vi "Build_Class_Tree.vi"() -> (2 "Root IDs":string[](array[string]), 3 "Map":map{string, cluster{string, variant}}(c390))   [LabVIEW 2025]
uses:
  <vilib>/_script/All Supported PropertiesOrMethods TypeDefs/ASC_ArrayOfUniqueIDStringParentIDStringName.ctl
  <vilib>/_script/All Supported PropertiesOrMethods TypeDefs/ASC_UniqueIDStringParentIDStringName.ctl
panel:
  out "size(s)":i32
  in  "All Types[]":T1=[{"Unique ID string"="3", "Parent ID string"="", "Class Name (unlocalized)"="Generic", "Class Name (localized)"="Generic"}, {"Unique ID string"="1", "Parent ID string"="", "Class Name (unlocalized)"="Application", "Class Name (localized)"="Application"}, {"Unique ID string"="2", "Parent ID string"="", "Class Name (unlocalized)"="VI", "Class Name (localized)"="VI"}, {"Unique ID string"="73", "Parent ID string"="", "Class Name (unlocalized)"="Project", "Class Name (localized)"="Project"}, {"Unique ID string"="74", "Parent ID string"="", "Class Name (unlocalized)"="ProjectItem", "Class Name (localized)"="ProjectItem"}, {"Unique ID string"="101", "Parent ID string"="2", "Class Name (unlocalized)"="PolymorphicVI", "Class Name (localized)"="PolymorphicVI"}, {"Unique ID string"="79", "Parent ID string"="2", "Class Name (unlocalized)"="FacadeVI", "Class Name (localized)"="FacadeVI"}, {"Unique ID string"="80", "Parent ID string"="74", "Class Name (unlocalized)"="Library", "Class Name (localized)"="Library"}, {"Unique ID string"="81", "Parent ID string"="", "Class Name (unlocalized)"="Variable", "Class Name (localized)"="Variable"}, {"Unique ID string"="82", "Parent ID string"="", "Class Name (unlocalized)"="TagSet", "Class Name (localized)"="TagSet"}, {"Unique ID string"="87", "Parent ID string"="2", "Class Name (unlocalized)"="MethodVI", "Class Name (localized)"="MethodVI"}, {"Unique ID string"="103", "Parent ID string"="80", "Class Name (unlocalized)"="XInterfaceLibrary", "Class Name (localized)"="XInterfaceLibrary"}, {"Unique ID string"="88", "Parent ID string"="103", "Class Name (unlocalized)"="XControlLibrary", "Class Name (localized)"="XControlLibrary"}, {"Unique ID string"="91", "Parent ID string"="", "Class Name (unlocalized)"="LVTarget", "Class Name (localized)"="LVTarget"}, {"Unique ID string"="93", "Parent ID string"="", "Class Name (unlocalized)"="Provider", "Class Name (localized)"="Provider"}, {"Unique ID string"="94", "Parent ID string"="", "Class Name (unlocalized)"="CopyOperation", "Class Name (localized)"="CopyOperation"}, {"Unique ID string"="95", "Parent ID string"="74", "Class Name (unlocalized)"="TargetItem", "Class Name (localized)"="TargetItem"}, {"Unique ID string"="96", "Parent ID string"="", "Class Name (unlocalized)"="ProjectItemType", "Class Name (localized)"="ProjectItemType"}, {"Unique ID string"="97", "Parent ID string"="", "Class Name (unlocalized)"="CopyItem", "Class Name (localized)"="CopyItem"}, {"Unique ID string"="98", "Parent ID string"="", "Class Name (unlocalized)"="CopyConflict", "Class Name (localized)"="CopyConflict"}, {"Unique ID string"="99", "Parent ID string"="", "Class Name (unlocalized)"="CopyExpert", "Class Name (localized)"="CopyExpert"}, {"Unique ID string"="123", "Parent ID string"="", "Class Name (unlocalized)"="Scene", "Class Name (localized)"="Scene"}, {"Unique ID string"="111", "Parent ID string"="123", "Class Name (unlocalized)"="SceneTexture", "Class Name (localized)"="SceneTexture"}, {"Unique ID string"="104", "Parent ID string"="123", "Class Name (unlocalized)"="SceneNode", "Class Name (localized)"="SceneNode"}, {"Unique ID string"="106", "Parent ID string"="104", "Class Name (unlocalized)"="SceneLight", "Class Name (localized)"="SceneLight"}, {"Unique ID string"="128", "Parent ID string"="123", "Class Name (unlocalized)"="SceneDrawable", "Class Name (localized)"="SceneDrawable"}, {"Unique ID string"="112", "Parent ID string"="128", "Class Name (unlocalized)"="SceneGeometry", "Class Name (localized)"="SceneGeometry"}, {"Unique ID string"="118", "Parent ID string"="112", "Class Name (unlocalized)"="SceneMesh", "Class Name (localized)"="SceneMesh"}, {"Unique ID string"="116", "Parent ID string"="112", "Class Name (unlocalized)"="SceneHeightField", "Class Name (localized)"="SceneHeightField"}, {"Unique ID string"="115", "Parent ID string"="112", "Class Name (unlocalized)"="SceneCylinder", "Class Name (localized)"="SceneCylinder"}, {"Unique ID string"="117", "Parent ID string"="112", "Class Name (unlocalized)"="SceneSphere", "Class Name (localized)"="SceneSphere"}, {"Unique ID string"="114", "Parent ID string"="112", "Class Name (unlocalized)"="SceneCone", "Class Name (localized)"="SceneCone"}, {"Unique ID string"="113", "Parent ID string"="112", "Class Name (unlocalized)"="SceneBox", "Class Name (localized)"="SceneBox"}, {"Unique ID string"="105", "Parent ID string"="104", "Class Name (unlocalized)"="SceneObject", "Class Name (localized)"="SceneObject"}, {"Unique ID string"="110", "Parent ID string"="104", "Class Name (unlocalized)"="SceneClipPlane", "Class Name (localized)"="SceneClipPlane"}, {"Unique ID string"="84", "Parent ID string"="123", "Class Name (unlocalized)"="SceneWindow", "Class Name (localized)"="SceneWindow"}, {"Unique ID string"="120", "Parent ID string"="74", "Class Name (unlocalized)"="PropertyFolder", "Class Name (localized)"="PropertyFolder"}, {"Unique ID string"="119", "Parent ID string"="120", "Class Name (unlocalized)"="XPropertyFolder", "Class Name (localized)"="XPropertyFolder"}, {"Unique ID string"="125", "Parent ID string"="74", "Class Name (unlocalized)"="LibraryData", "Class Name (localized)"="LibraryData"}, {"Unique ID string"="129", "Parent ID string"="128", "Class Name (unlocalized)"="SceneText", "Class Name (localized)"="SceneText"}, {"Unique ID string"="62", "Parent ID string"="2", "Class Name (unlocalized)"="SubsystemVI", "Class Name (localized)"="SubsystemVI"}, {"Unique ID string"="133", "Parent ID string"="", "Class Name (unlocalized)"="ProjectFilesViewItem", "Class Name (localized)"="ProjectFilesViewItem"}, {"Unique ID string"="134", "Parent ID string"="74", "Class Name (unlocalized)"="LVClassPropDefFolder", "Class Name (localized)"="LVClassPropDefFolder"}, {"Unique ID string"="36", "Parent ID string"="3", "Class Name (unlocalized)"="GObject", "Class Name (localized)"="GObject"}, {"Unique ID string"="37", "Parent ID string"="3", "Class Name (unlocalized)"="Plot", "Class Name (localized)"="Plot"}, {"Unique ID string"="38", "Parent ID string"="3", "Class Name (unlocalized)"="Cursor", "Class Name (localized)"="Cursor"}, {"Unique ID string"="4", "Parent ID string"="36", "Class Name (unlocalized)"="Decoration", "Class Name (localized)"="Decoration"}, {"Unique ID string"="5", "Parent ID string"="4", "Class Name (unlocalized)"="Text", "Class Name (localized)"="Text"}, {"Unique ID string"="39", "Parent ID string"="5", "Class Name (unlocalized)"="NumericText", "Class Name (localized)"="NumericText"}, {"Unique ID string"="40", "Parent ID string"="36", "Class Name (unlocalized)"="Scale", "Class Name (localized)"="Scale"}, {"Unique ID string"="41", "Parent ID string"="40", "Class Name (unlocalized)"="ColorScale", "Class Name (localized)"="ColorScale"}, {"Unique ID string"="42", "Parent ID string"="40", "Class Name (unlocalized)"="GraphScale", "Class Name (localized)"="GraphScale"}, {"Unique ID string"="43", "Parent ID string"="40", "Class Name (unlocalized)"="ColorGraphScale", "Class Name (localized)"="ColorGraphScale"}, {"Unique ID string"="6", "Parent ID string"="36", "Class Name (unlocalized)"="Control", "Class Name (localized)"="Control"}, {"Unique ID string"="7", "Parent ID string"="6", "Class Name (unlocalized)"="ColorBox", "Class Name (localized)"="ColorBox"}, {"Unique ID string"="8", "Parent ID string"="6", "Class Name (unlocalized)"="Boolean", "Class Name (localized)"="Boolean"}, {"Unique ID string"="9", "Parent ID string"="6", "Class Name (unlocalized)"="RefNum", "Class Name (localized)"="RefNum"}, {"Unique ID string"="44", "Parent ID string"="9", "Class Name (unlocalized)"="TypedRefNum", "Class Name (localized)"="TypedRefNum"}, {"Unique ID string"="10", "Parent ID string"="6", "Class Name (unlocalized)"="LVVariant", "Class Name (localized)"="LVVariant"}, {"Unique ID string"="11", "Parent ID string"="6", "Class Name (unlocalized)"="Path", "Class Name (localized)"="Path"}, {"Unique ID string"="12", "Parent ID string"="6", "Class Name (unlocalized)"="ListBox", "Class Name (localized)"="ListBox"}, {"Unique ID string"="13", "Parent ID string"="6", "Class Name (unlocalized)"="Table", "Class Name (localized)"="Table"}, {"Unique ID string"="14", "Parent ID string"="6", "Class Name (unlocalized)"="Array", "Class Name (localized)"="Array"}, {"Unique ID string"="15", "Parent ID string"="6", "Class Name (unlocalized)"="Picture", "Class Name (localized)"="Picture"}, {"Unique ID string"="16", "Parent ID string"="6", "Class Name (unlocalized)"="ActiveXContainer", "Class Name (localized)"="ActiveXContainer"}, {"Unique ID string"="17", "Parent ID string"="6", "Class Name (unlocalized)"="Numeric", "Class Name (localized)"="Numeric"}, {"Unique ID string"="18", "Parent ID string"="17", "Class Name (unlocalized)"="Digital", "Class Name (localized)"="Digital"}, {"Unique ID string"="19", "Parent ID string"="17", "Class Name (unlocalized)"="NamedNumeric", "Class Name (localized)"="NamedNumeric"}, {"Unique ID string"="35", "Parent ID string"="19", "Class Name (unlocalized)"="Enum", "Class Name (localized)"="Enum"}, {"Unique ID string"="34", "Parent ID string"="19", "Class Name (unlocalized)"="Ring", "Class Name (localized)"="Ring"}, {"Unique ID string"="20", "Parent ID string"="17", "Class Name (unlocalized)"="ColorRamp", "Class Name (localized)"="ColorRamp"}, {"Unique ID string"="33", "Parent ID string"="17", "Class Name (unlocalized)"="NumericWithScale", "Class Name (localized)"="NumericWithScale"}, {"Unique ID string"="21", "Parent ID string"="33", "Class Name (unlocalized)"="Slide", "Class Name (localized)"="Slide"}, {"Unique ID string"="32", "Parent ID string"="33", "Class Name (unlocalized)"="Knob", "Class Name (localized)"="Knob"}, {"Unique ID string"="22", "Parent ID string"="6", "Class Name (unlocalized)"="GraphChart", "Class Name (localized)"="GraphChart"}, {"Unique ID string"="23", "Parent ID string"="22", "Class Name (unlocalized)"="WaveformChart", "Class Name (localized)"="WaveformChart"}, {"Unique ID string"="24", "Parent ID string"="22", "Class Name (unlocalized)"="WaveformGraph", "Class Name (localized)"="WaveformGraph"}, {"Unique ID string"="25", "Parent ID string"="22", "Class Name (unlocalized)"="IntensityChart", "Class Name (localized)"="IntensityChart"}, {"Unique ID string"="26", "Parent ID string"="22", "Class Name (unlocalized)"="IntensityGraph", "Class Name (localized)"="IntensityGraph"}, {"Unique ID string"="27", "Parent ID string"="6", "Class Name (unlocalized)"="String", "Class Name (localized)"="String"}, {"Unique ID string"="28", "Parent ID string"="6", "Class Name (unlocalized)"="IOName", "Class Name (localized)"="IOName"}, {"Unique ID string"="29", "Parent ID string"="27", "Class Name (unlocalized)"="ComboBox", "Class Name (localized)"="ComboBox"}, {"Unique ID string"="30", "Parent ID string"="6", "Class Name (unlocalized)"="Cluster", "Class Name (localized)"="Cluster"}, {"Unique ID string"="31", "Parent ID string"="36", "Class Name (unlocalized)"="Panel", "Class Name (localized)"="Panel"}, {"Unique ID string"="46", "Parent ID string"="6", "Class Name (unlocalized)"="MulticolumnListbox", "Class Name (localized)"="MulticolumnListbox"}, {"Unique ID string"="47", "Parent ID string"="6", "Class Name (unlocalized)"="WaveformData", "Class Name (localized)"="WaveformData"}, {"Unique ID string"="48", "Parent ID string"="28", "Class Name (unlocalized)"="DSCTag", "Class Name (localized)"="DSCTag"}, {"Unique ID string"="49", "Parent ID string"="28", "Class Name (unlocalized)"="DAQChannelName", "Class Name (localized)"="DAQChannelName"}, {"Unique ID string"="50", "Parent ID string"="28", "Class Name (unlocalized)"="VISAResourceName", "Class Name (localized)"="VISAResourceName"}, {"Unique ID string"="51", "Parent ID string"="28", "Class Name (unlocalized)"="IVILogicalName", "Class Name (localized)"="IVILogicalName"}, {"Unique ID string"="52", "Parent ID string"="40", "Class Name (unlocalized)"="SlideScale", "Class Name (localized)"="SlideScale"}, {"Unique ID string"="53", "Parent ID string"="6", "Class Name (unlocalized)"="PageSelector", "Class Name (localized)"="PageSelector"}, {"Unique ID string"="54", "Parent ID string"="3", "Class Name (unlocalized)"="Page", "Class Name (localized)"="Page"}, {"Unique ID string"="55", "Parent ID string"="53", "Class Name (unlocalized)"="TabControl", "Class Name (localized)"="TabControl"}, {"Unique ID string"="56", "Parent ID string"="3", "Class Name (unlocalized)"="ConnectorPane", "Class Name (localized)"="ConnectorPane"}, {"Unique ID string"="57", "Parent ID string"="28", "Class Name (unlocalized)"="DAQmxName", "Class Name (localized)"="DAQmxName"}, {"Unique ID string"="59", "Parent ID string"="9", "Class Name (unlocalized)"="LVObjectRefNum", "Class Name (localized)"="LVObjectRefNum"}, {"Unique ID string"="58", "Parent ID string"="59", "Class Name (unlocalized)"="VIRefNum", "Class Name (localized)"="VIRefNum"}, {"Unique ID string"="60", "Parent ID string"="6", "Class Name (unlocalized)"="AbsTime", "Class Name (localized)"="AbsTime"}, {"Unique ID string"="61", "Parent ID string"="6", "Class Name (unlocalized)"="DigitalTable", "Class Name (localized)"="DigitalTable"}, {"Unique ID string"="66", "Parent ID string"="6", "Class Name (unlocalized)"="TreeControl", "Class Name (localized)"="TreeControl"}, {"Unique ID string"="67", "Parent ID string"="28", "Class Name (unlocalized)"="GenClassTagRef", "Class Name (localized)"="GenClassTagRef"}, {"Unique ID string"="68", "Parent ID string"="9", "Class Name (unlocalized)"="GenClassRef", "Class Name (localized)"="GenClassRef"}, {"Unique ID string"="65", "Parent ID string"="6", "Class Name (unlocalized)"="SubPanel", "Class Name (localized)"="SubPanel"}, {"Unique ID string"="69", "Parent ID string"="41", "Class Name (unlocalized)"="RotaryColorScale", "Class Name (localized)"="RotaryColorScale"}, {"Unique ID string"="70", "Parent ID string"="6", "Class Name (unlocalized)"="PlugInControl", "Class Name (localized)"="PlugInControl"}, {"Unique ID string"="71", "Parent ID string"="6", "Class Name (unlocalized)"="PlugInDDODummyContainer", "Class Name (localized)"="PlugInDDODummyContainer"}, {"Unique ID string"="122", "Parent ID string"="28", "Class Name (unlocalized)"="GenClassTagFlatRef", "Class Name (localized)"="GenClassTagFlatRef"}, {"Unique ID string"="72", "Parent ID string"="30", "Class Name (unlocalized)"="RadioButtonsControl", "Class Name (localized)"="RadioButtonsControl"}, {"Unique ID string"="75", "Parent ID string"="36", "Class Name (unlocalized)"="Pane", "Class Name (localized)"="Pane"}, {"Unique ID string"="77", "Parent ID string"="74", "Class Name (unlocalized)"="BuildSpecification", "Class Name (localized)"="BuildSpecification"}, {"Unique ID string"="78", "Parent ID string"="6", "Class Name (unlocalized)"="Pixmap", "Class Name (localized)"="Pixmap"}, {"Unique ID string"="83", "Parent ID string"="24", "Class Name (unlocalized)"="XYGraph", "Class Name (localized)"="XYGraph"}, {"Unique ID string"="76", "Parent ID string"="36", "Class Name (unlocalized)"="Splitter", "Class Name (localized)"="Splitter"}, {"Unique ID string"="85", "Parent ID string"="80", "Class Name (unlocalized)"="LVClassLibrary", "Class Name (localized)"="LVClassLibrary"}, {"Unique ID string"="89", "Parent ID string"="103", "Class Name (unlocalized)"="XNodeLibrary", "Class Name (localized)"="XNodeLibrary"}, {"Unique ID string"="90", "Parent ID string"="6", "Class Name (unlocalized)"="Scrollbar", "Class Name (localized)"="Scrollbar"}, {"Unique ID string"="92", "Parent ID string"="22", "Class Name (unlocalized)"="MixedSignalGraph", "Class Name (localized)"="MixedSignalGraph"}, {"Unique ID string"="100", "Parent ID string"="6", "Class Name (unlocalized)"="SceneGraphDisplay", "Class Name (localized)"="SceneGraphDisplay"}, {"Unique ID string"="102", "Parent ID string"="6", "Class Name (unlocalized)"="LabVIEWClassControl", "Class Name (localized)"="LabVIEWClassControl"}, {"Unique ID string"="121", "Parent ID string"="24", "Class Name (unlocalized)"="DigitalGraph", "Class Name (localized)"="DigitalGraph"}, {"Unique ID string"="126", "Parent ID string"="80", "Class Name (unlocalized)"="StatechartLibrary", "Class Name (localized)"="StatechartLibrary"}, {"Unique ID string"="127", "Parent ID string"="6", "Class Name (unlocalized)"="MixedCheckbox", "Class Name (localized)"="MixedCheckbox"}, {"Unique ID string"="130", "Parent ID string"="6", "Class Name (unlocalized)"="MultiSegmentPipe", "Class Name (localized)"="MultiSegmentPipe"}, {"Unique ID string"="131", "Parent ID string"="3", "Class Name (unlocalized)"="Bus", "Class Name (localized)"="Bus"}, {"Unique ID string"="132", "Parent ID string"="6", "Class Name (unlocalized)"="StubDDO", "Class Name (localized)"="StubDDO"}, {"Unique ID string"="135", "Parent ID string"="44", "Class Name (unlocalized)"="DataValRefNum", "Class Name (localized)"="DataValRefNum"}, {"Unique ID string"="136", "Parent ID string"="6", "Class Name (unlocalized)"="Set", "Class Name (localized)"="Set"}, {"Unique ID string"="137", "Parent ID string"="6", "Class Name (unlocalized)"="Map", "Class Name (localized)"="Map"}, {"Unique ID string"="16503", "Parent ID string"="36", "Class Name (unlocalized)"="AbstractDiagram", "Class Name (localized)"="AbstractDiagram"}, {"Unique ID string"="16384", "Parent ID string"="16503", "Class Name (unlocalized)"="Diagram", "Class Name (localized)"="Diagram"}, {"Unique ID string"="16423", "Parent ID string"="16384", "Class Name (unlocalized)"="TopLevelDiagram", "Class Name (localized)"="TopLevelDiagram"}, {"Unique ID string"="16385", "Parent ID string"="36", "Class Name (unlocalized)"="Terminal", "Class Name (localized)"="Terminal"}, {"Unique ID string"="16386", "Parent ID string"="36", "Class Name (unlocalized)"="Constant", "Class Name (localized)"="Constant"}, {"Unique ID string"="16387", "Parent ID string"="16386", "Class Name (unlocalized)"="PathConstant", "Class Name (localized)"="PathConstant"}, {"Unique ID string"="16388", "Parent ID string"="16386", "Class Name (unlocalized)"="ArrayConstant", "Class Name (localized)"="ArrayConstant"}, {"Unique ID string"="16389", "Parent ID string"="16386", "Class Name (unlocalized)"="NumericConstant", "Class Name (localized)"="NumericConstant"}, {"Unique ID string"="16390", "Parent ID string"="16389", "Class Name (unlocalized)"="DigitalNumericConstant", "Class Name (localized)"="DigitalNumericConstant"}, {"Unique ID string"="16391", "Parent ID string"="16389", "Class Name (unlocalized)"="NamedNumericConstant", "Class Name (localized)"="NamedNumericConstant"}, {"Unique ID string"="16424", "Parent ID string"="16391", "Class Name (unlocalized)"="RingConstant", "Class Name (localized)"="RingConstant"}, {"Unique ID string"="16425", "Parent ID string"="16391", "Class Name (unlocalized)"="EnumConstant", "Class Name (localized)"="EnumConstant"}, {"Unique ID string"="16392", "Parent ID string"="16386", "Class Name (unlocalized)"="StringConstant", "Class Name (localized)"="StringConstant"}, {"Unique ID string"="16393", "Parent ID string"="16386", "Class Name (unlocalized)"="ClusterConstant", "Class Name (localized)"="ClusterConstant"}, {"Unique ID string"="16394", "Parent ID string"="16386", "Class Name (unlocalized)"="FixedConstant", "Class Name (localized)"="FixedConstant"}, {"Unique ID string"="16422", "Parent ID string"="16386", "Class Name (unlocalized)"="BooleanConstant", "Class Name (localized)"="BooleanConstant"}, {"Unique ID string"="16395", "Parent ID string"="16385", "Class Name (unlocalized)"="ControlTerminal", "Class Name (localized)"="ControlTerminal"}, {"Unique ID string"="16396", "Parent ID string"="36", "Class Name (unlocalized)"="FormulaParameter", "Class Name (localized)"="FormulaParameter"}, {"Unique ID string"="16426", "Parent ID string"="36", "Class Name (unlocalized)"="Tunnel", "Class Name (localized)"="Tunnel"}, {"Unique ID string"="16427", "Parent ID string"="16426", "Class Name (unlocalized)"="LoopTunnel", "Class Name (localized)"="LoopTunnel"}, {"Unique ID string"="16399", "Parent ID string"="16426", "Class Name (unlocalized)"="RightShiftRegister", "Class Name (localized)"="RightShiftRegister"}, {"Unique ID string"="16428", "Parent ID string"="36", "Class Name (unlocalized)"="SequenceLocal", "Class Name (localized)"="SequenceLocal"}, {"Unique ID string"="16421", "Parent ID string"="36", "Class Name (unlocalized)"="Node", "Class Name (localized)"="Node"}, {"Unique ID string"="16397", "Parent ID string"="16421", "Class Name (unlocalized)"="Global", "Class Name (localized)"="Global"}, {"Unique ID string"="16398", "Parent ID string"="16421", "Class Name (unlocalized)"="Local", "Class Name (localized)"="Local"}, {"Unique ID string"="16400", "Parent ID string"="16421", "Class Name (unlocalized)"="Function", "Class Name (localized)"="Function"}, {"Unique ID string"="16429", "Parent ID string"="16400", "Class Name (unlocalized)"="Comparison", "Class Name (localized)"="Comparison"}, {"Unique ID string"="16430", "Parent ID string"="16400", "Class Name (unlocalized)"="ReadWriteFile", "Class Name (localized)"="ReadWriteFile"}, {"Unique ID string"="16431", "Parent ID string"="16400", "Class Name (unlocalized)"="TypeCast", "Class Name (localized)"="TypeCast"}, {"Unique ID string"="16432", "Parent ID string"="16400", "Class Name (unlocalized)"="FlattenUnflattenString", "Class Name (localized)"="FlattenUnflattenString"}, {"Unique ID string"="16433", "Parent ID string"="16400", "Class Name (unlocalized)"="GPIBReadWrite", "Class Name (localized)"="GPIBReadWrite"}, {"Unique ID string"="16401", "Parent ID string"="16421", "Class Name (unlocalized)"="SubVI", "Class Name (localized)"="SubVI"}, {"Unique ID string"="16402", "Parent ID string"="16421", "Class Name (unlocalized)"="CallByRef", "Class Name (localized)"="CallByRef"}, {"Unique ID string"="16403", "Parent ID string"="16421", "Class Name (unlocalized)"="UnitCast", "Class Name (localized)"="UnitCast"}, {"Unique ID string"="16404", "Parent ID string"="16421", "Class Name (unlocalized)"="Structure", "Class Name (localized)"="Structure"}, {"Unique ID string"="16405", "Parent ID string"="16404", "Class Name (unlocalized)"="Loop", "Class Name (localized)"="Loop"}, {"Unique ID string"="16434", "Parent ID string"="16405", "Class Name (unlocalized)"="ForLoop", "Class Name (localized)"="ForLoop"}, {"Unique ID string"="16435", "Parent ID string"="16405", "Class Name (unlocalized)"="WhileLoop", "Class Name (localized)"="WhileLoop"}, {"Unique ID string"="16406", "Parent ID string"="16404", "Class Name (unlocalized)"="MultiFrameStructure", "Class Name (localized)"="MultiFrameStructure"}, {"Unique ID string"="16407", "Parent ID string"="16406", "Class Name (unlocalized)"="Sequence", "Class Name (localized)"="Sequence"}, {"Unique ID string"="16408", "Parent ID string"="16406", "Class Name (unlocalized)"="CaseStructure", "Class Name (localized)"="CaseStructure"}, {"Unique ID string"="16409", "Parent ID string"="16421", "Class Name (unlocalized)"="Formula", "Class Name (localized)"="Formula"}, {"Unique ID string"="16436", "Parent ID string"="16409", "Class Name (unlocalized)"="ScriptNode", "Class Name (localized)"="ScriptNode"}, {"Unique ID string"="16437", "Parent ID string"="16400", "Class Name (unlocalized)"="ArrayToCluster", "Class Name (localized)"="ArrayToCluster"}, {"Unique ID string"="16410", "Parent ID string"="16421", "Class Name (unlocalized)"="GrowableFunction", "Class Name (localized)"="GrowableFunction"}, {"Unique ID string"="16411", "Parent ID string"="16410", "Class Name (unlocalized)"="BuildClusterArray", "Class Name (localized)"="BuildClusterArray"}, {"Unique ID string"="16412", "Parent ID string"="16410", "Class Name (unlocalized)"="CompoundArithmetic", "Class Name (localized)"="CompoundArithmetic"}, {"Unique ID string"="16413", "Parent ID string"="16410", "Class Name (unlocalized)"="IndexArray", "Class Name (localized)"="IndexArray"}, {"Unique ID string"="16416", "Parent ID string"="16410", "Class Name (unlocalized)"="CIN", "Class Name (localized)"="CIN"}, {"Unique ID string"="16417", "Parent ID string"="16410", "Class Name (unlocalized)"="CallLibrary", "Class Name (localized)"="CallLibrary"}, {"Unique ID string"="16438", "Parent ID string"="16410", "Class Name (unlocalized)"="FormatScanString", "Class Name (localized)"="FormatScanString"}, {"Unique ID string"="16418", "Parent ID string"="16410", "Class Name (unlocalized)"="ObjectFunction", "Class Name (localized)"="ObjectFunction"}, {"Unique ID string"="16419", "Parent ID string"="16418", "Class Name (unlocalized)"="Property", "Class Name (localized)"="Property"}, {"Unique ID string"="16420", "Parent ID string"="16418", "Class Name (unlocalized)"="Invoke", "Class Name (localized)"="Invoke"}, {"Unique ID string"="16439", "Parent ID string"="36", "Class Name (unlocalized)"="Wire", "Class Name (localized)"="Wire"}, {"Unique ID string"="16440", "Parent ID string"="3", "Class Name (unlocalized)"="Probe", "Class Name (localized)"="Probe"}, {"Unique ID string"="16441", "Parent ID string"="16385", "Class Name (unlocalized)"="InnerTerminal", "Class Name (localized)"="InnerTerminal"}, {"Unique ID string"="16442", "Parent ID string"="16426", "Class Name (unlocalized)"="LeftShiftRegister", "Class Name (localized)"="LeftShiftRegister"}, {"Unique ID string"="16443", "Parent ID string"="16401", "Class Name (unlocalized)"="PolymorphicSubVI", "Class Name (localized)"="PolymorphicSubVI"}, {"Unique ID string"="16444", "Parent ID string"="36", "Class Name (unlocalized)"="PropertyItem", "Class Name (localized)"="PropertyItem"}, {"Unique ID string"="16445", "Parent ID string"="16386", "Class Name (unlocalized)"="IONameConstant", "Class Name (localized)"="IONameConstant"}, {"Unique ID string"="16446", "Parent ID string"="16445", "Class Name (unlocalized)"="DSCTagConstant", "Class Name (localized)"="DSCTagConstant"}, {"Unique ID string"="16447", "Parent ID string"="16445", "Class Name (unlocalized)"="DAQChannelNameConstant", "Class Name (localized)"="DAQChannelNameConstant"}, {"Unique ID string"="16448", "Parent ID string"="16445", "Class Name (unlocalized)"="VISAResourceNameConstant", "Class Name (localized)"="VISAResourceNameConstant"}, {"Unique ID string"="16449", "Parent ID string"="16445", "Class Name (unlocalized)"="IVILogicalNameConstant", "Class Name (localized)"="IVILogicalNameConstant"}, {"Unique ID string"="16450", "Parent ID string"="16386", "Class Name (unlocalized)"="ColorBoxConstant", "Class Name (localized)"="ColorBoxConstant"}, {"Unique ID string"="16451", "Parent ID string"="16421", "Class Name (unlocalized)"="ControlReferenceConstant", "Class Name (localized)"="ControlReferenceConstant"}, {"Unique ID string"="16453", "Parent ID string"="16401", "Class Name (unlocalized)"="ConfNode", "Class Name (localized)"="ConfNode"}, {"Unique ID string"="16456", "Parent ID string"="16385", "Class Name (unlocalized)"="OuterTerminal", "Class Name (localized)"="OuterTerminal"}, {"Unique ID string"="16457", "Parent ID string"="16445", "Class Name (unlocalized)"="DAQmxNameConstant", "Class Name (localized)"="DAQmxNameConstant"}, {"Unique ID string"="16458", "Parent ID string"="16406", "Class Name (unlocalized)"="EventStructure", "Class Name (localized)"="EventStructure"}, {"Unique ID string"="16459", "Parent ID string"="36", "Class Name (unlocalized)"="FlatSequence", "Class Name (localized)"="FlatSequence"}, {"Unique ID string"="16460", "Parent ID string"="16445", "Class Name (unlocalized)"="GenClassTagRefConstant", "Class Name (localized)"="GenClassTagRefConstant"}, {"Unique ID string"="16461", "Parent ID string"="16386", "Class Name (unlocalized)"="AbsTimeConstant", "Class Name (localized)"="AbsTimeConstant"}, {"Unique ID string"="16462", "Parent ID string"="16407", "Class Name (unlocalized)"="ExternalNode", "Class Name (localized)"="ExternalNode"}, {"Unique ID string"="16466", "Parent ID string"="16392", "Class Name (unlocalized)"="ComboBoxConstant", "Class Name (localized)"="ComboBoxConstant"}, {"Unique ID string"="16463", "Parent ID string"="3", "Class Name (unlocalized)"="SubWizard", "Class Name (localized)"="SubWizard"}, {"Unique ID string"="16455", "Parent ID string"="16463", "Class Name (unlocalized)"="StateDiagramWizard", "Class Name (localized)"="StateDiagramWizard"}, {"Unique ID string"="16464", "Parent ID string"="16396", "Class Name (unlocalized)"="ScriptNodeParameter", "Class Name (localized)"="ScriptNodeParameter"}, {"Unique ID string"="16465", "Parent ID string"="16421", "Class Name (unlocalized)"="StaticVIReference", "Class Name (localized)"="StaticVIReference"}, {"Unique ID string"="16467", "Parent ID string"="16435", "Class Name (unlocalized)"="TimedLoop", "Class Name (localized)"="TimedLoop"}, {"Unique ID string"="16470", "Parent ID string"="16445", "Class Name (unlocalized)"="GenClassTagFlatRefConstant", "Class Name (localized)"="GenClassTagFlatRefConstant"}, {"Unique ID string"="16472", "Parent ID string"="16384", "Class Name (unlocalized)"="SimDiagram", "Class Name (localized)"="SimDiagram"}, {"Unique ID string"="16473", "Parent ID string"="16384", "Class Name (unlocalized)"="CompanionDiagram", "Class Name (localized)"="CompanionDiagram"}, {"Unique ID string"="16474", "Parent ID string"="16404", "Class Name (unlocalized)"="SimulationNode", "Class Name (localized)"="SimulationNode"}, {"Unique ID string"="16476", "Parent ID string"="16410", "Class Name (unlocalized)"="Bundler", "Class Name (localized)"="Bundler"}, {"Unique ID string"="16477", "Parent ID string"="16410", "Class Name (unlocalized)"="Unbundler", "Class Name (localized)"="Unbundler"}, {"Unique ID string"="16414", "Parent ID string"="16476", "Class Name (unlocalized)"="BuildArray", "Class Name (localized)"="BuildArray"}, {"Unique ID string"="16415", "Parent ID string"="16476", "Class Name (unlocalized)"="NamedBundler", "Class Name (localized)"="NamedBundler"}, {"Unique ID string"="16475", "Parent ID string"="36", "Class Name (unlocalized)"="SimulationDCO", "Class Name (localized)"="SimulationDCO"}, {"Unique ID string"="16478", "Parent ID string"="16477", "Class Name (unlocalized)"="NamedUnbundler", "Class Name (localized)"="NamedUnbundler"}, {"Unique ID string"="16479", "Parent ID string"="3", "Class Name (unlocalized)"="FlatSequenceFrame", "Class Name (localized)"="FlatSequenceFrame"}, {"Unique ID string"="16480", "Parent ID string"="36", "Class Name (unlocalized)"="FlatSequenceInnerTunnel", "Class Name (localized)"="FlatSequenceInnerTunnel"}, {"Unique ID string"="16481", "Parent ID string"="36", "Class Name (unlocalized)"="FlatSequenceOuterTunnel", "Class Name (localized)"="FlatSequenceOuterTunnel"}, {"Unique ID string"="16482", "Parent ID string"="16386", "Class Name (unlocalized)"="RefNumConstant", "Class Name (localized)"="RefNumConstant"}, {"Unique ID string"="16452", "Parent ID string"="16482", "Class Name (unlocalized)"="ClassSpecifierConstant", "Class Name (localized)"="ClassSpecifierConstant"}, {"Unique ID string"="16483", "Parent ID string"="16432", "Class Name (unlocalized)"="FlattenString", "Class Name (localized)"="FlattenString"}, {"Unique ID string"="16484", "Parent ID string"="36", "Class Name (unlocalized)"="PolymorphicVISelector", "Class Name (localized)"="PolymorphicVISelector"}, {"Unique ID string"="16485", "Parent ID string"="16421", "Class Name (unlocalized)"="XNode", "Class Name (localized)"="XNode"}, {"Unique ID string"="16486", "Parent ID string"="16525", "Class Name (unlocalized)"="SelectorTunnel", "Class Name (localized)"="SelectorTunnel"}, {"Unique ID string"="16487", "Parent ID string"="16406", "Class Name (unlocalized)"="DisableStructure", "Class Name (localized)"="DisableStructure"}, {"Unique ID string"="16491", "Parent ID string"="36", "Class Name (unlocalized)"="SynchronousDataFlowDCO", "Class Name (localized)"="SynchronousDataFlowDCO"}, {"Unique ID string"="16490", "Parent ID string"="16404", "Class Name (unlocalized)"="SynchronousDataFlowNode", "Class Name (localized)"="SynchronousDataFlowNode"}, {"Unique ID string"="16489", "Parent ID string"="16384", "Class Name (unlocalized)"="SDF Companion Diagram", "Class Name (localized)"="SDF Companion Diagram"}, {"Unique ID string"="16488", "Parent ID string"="16384", "Class Name (unlocalized)"="SDFDiagram", "Class Name (localized)"="SDFDiagram"}, {"Unique ID string"="16492", "Parent ID string"="16400", "Class Name (unlocalized)"="FileDialog", "Class Name (localized)"="FileDialog"}, {"Unique ID string"="16498", "Parent ID string"="16463", "Class Name (unlocalized)"="CodeWizard", "Class Name (localized)"="CodeWizard"}, {"Unique ID string"="16454", "Parent ID string"="3", "Class Name (unlocalized)"="MasterWizard", "Class Name (localized)"="MasterWizard"}, {"Unique ID string"="16494", "Parent ID string"="16479", "Class Name (unlocalized)"="TimeSequenceFrame", "Class Name (localized)"="TimeSequenceFrame"}, {"Unique ID string"="16495", "Parent ID string"="16459", "Class Name (unlocalized)"="TimeFlatSequence", "Class Name (localized)"="TimeFlatSequence"}, {"Unique ID string"="16496", "Parent ID string"="16404", "Class Name (unlocalized)"="TimedSequence", "Class Name (localized)"="TimedSequence"}, {"Unique ID string"="16493", "Parent ID string"="36", "Class Name (unlocalized)"="TimedStructDCO", "Class Name (localized)"="TimedStructDCO"}, {"Unique ID string"="16497", "Parent ID string"="16485", "Class Name (unlocalized)"="XDataNode", "Class Name (localized)"="XDataNode"}, {"Unique ID string"="16499", "Parent ID string"="16409", "Class Name (unlocalized)"="MathScriptNode", "Class Name (localized)"="MathScriptNode"}, {"Unique ID string"="16500", "Parent ID string"="16396", "Class Name (unlocalized)"="MathScriptNodeParameter", "Class Name (localized)"="MathScriptNodeParameter"}, {"Unique ID string"="16501", "Parent ID string"="16386", "Class Name (unlocalized)"="LabVIEWClassConstant", "Class Name (localized)"="LabVIEWClassConstant"}, {"Unique ID string"="16502", "Parent ID string"="16503", "Class Name (unlocalized)"="MathDiagram", "Class Name (localized)"="MathDiagram"}, {"Unique ID string"="16505", "Parent ID string"="16418", "Class Name (unlocalized)"="Constructor", "Class Name (localized)"="Constructor"}, {"Unique ID string"="16537", "Parent ID string"="16404", "Class Name (unlocalized)"="StatechartStructureNode", "Class Name (localized)"="StatechartStructureNode"}, {"Unique ID string"="16510", "Parent ID string"="16537", "Class Name (unlocalized)"="JoinNode", "Class Name (localized)"="JoinNode"}, {"Unique ID string"="16509", "Parent ID string"="16537", "Class Name (unlocalized)"="ForkNode", "Class Name (localized)"="ForkNode"}, {"Unique ID string"="16508", "Parent ID string"="16537", "Class Name (unlocalized)"="StateNode", "Class Name (localized)"="StateNode"}, {"Unique ID string"="16507", "Parent ID string"="16537", "Class Name (unlocalized)"="JunctionNode", "Class Name (localized)"="JunctionNode"}, {"Unique ID string"="16506", "Parent ID string"="16537", "Class Name (unlocalized)"="RegionNode", "Class Name (localized)"="RegionNode"}, {"Unique ID string"="16511", "Parent ID string"="16384", "Class Name (unlocalized)"="ScDiagram", "Class Name (localized)"="ScDiagram"}, {"Unique ID string"="16512", "Parent ID string"="16421", "Class Name (unlocalized)"="SharedVariableNode", "Class Name (localized)"="SharedVariableNode"}, {"Unique ID string"="16514", "Parent ID string"="16385", "Class Name (unlocalized)"="ParameterTerminal", "Class Name (localized)"="ParameterTerminal"}, {"Unique ID string"="16515", "Parent ID string"="16514", "Class Name (unlocalized)"="OverridableParameterTerminal", "Class Name (localized)"="OverridableParameterTerminal"}, {"Unique ID string"="16516", "Parent ID string"="16404", "Class Name (unlocalized)"="InPlaceElementStructure", "Class Name (localized)"="InPlaceElementStructure"}, {"Unique ID string"="16517", "Parent ID string"="16421", "Class Name (unlocalized)"="InPlaceBorderNode", "Class Name (localized)"="InPlaceBorderNode"}, {"Unique ID string"="16521", "Parent ID string"="16517", "Class Name (unlocalized)"="InPlaceElementNode", "Class Name (localized)"="InPlaceElementNode"}, {"Unique ID string"="16520", "Parent ID string"="16517", "Class Name (unlocalized)"="InPlaceVariantNode", "Class Name (localized)"="InPlaceVariantNode"}, {"Unique ID string"="16518", "Parent ID string"="16517", "Class Name (unlocalized)"="InPlaceArrayNode", "Class Name (localized)"="InPlaceArrayNode"}, {"Unique ID string"="16519", "Parent ID string"="16517", "Class Name (unlocalized)"="InPlaceClusterNode", "Class Name (localized)"="InPlaceClusterNode"}, {"Unique ID string"="16522", "Parent ID string"="16421", "Class Name (unlocalized)"="FeedbackNode", "Class Name (localized)"="FeedbackNode"}, {"Unique ID string"="16523", "Parent ID string"="16421", "Class Name (unlocalized)"="MathScriptCallByRef", "Class Name (localized)"="MathScriptCallByRef"}, {"Unique ID string"="16524", "Parent ID string"="16517", "Class Name (unlocalized)"="InPlaceDataValRefNode", "Class Name (localized)"="InPlaceDataValRefNode"}, {"Unique ID string"="16525", "Parent ID string"="16426", "Class Name (unlocalized)"="ConditionalTunnel", "Class Name (localized)"="ConditionalTunnel"}, {"Unique ID string"="16526", "Parent ID string"="16401", "Class Name (unlocalized)"="AbstractDynamicDispatch", "Class Name (localized)"="AbstractDynamicDispatch"}, {"Unique ID string"="16527", "Parent ID string"="16526", "Class Name (unlocalized)"="DynamicDispatchSubVI", "Class Name (localized)"="DynamicDispatchSubVI"}, {"Unique ID string"="16528", "Parent ID string"="16526", "Class Name (unlocalized)"="CallParentNode", "Class Name (localized)"="CallParentNode"}, {"Unique ID string"="16504", "Parent ID string"="16409", "Class Name (unlocalized)"="InlineCNode", "Class Name (localized)"="InlineCNode"}, {"Unique ID string"="16529", "Parent ID string"="16482", "Class Name (unlocalized)"="GenClassRefConst", "Class Name (localized)"="GenClassRefConst"}, {"Unique ID string"="16530", "Parent ID string"="16517", "Class Name (unlocalized)"="InPlaceArraySplitNode", "Class Name (localized)"="InPlaceArraySplitNode"}, {"Unique ID string"="16531", "Parent ID string"="16421", "Class Name (unlocalized)"="SharedVariableDynamicOpen", "Class Name (localized)"="SharedVariableDynamicOpen"}, {"Unique ID string"="16532", "Parent ID string"="16421", "Class Name (unlocalized)"="SharedVariableDynamicRead", "Class Name (localized)"="SharedVariableDynamicRead"}, {"Unique ID string"="16533", "Parent ID string"="16421", "Class Name (unlocalized)"="SharedVariableDynamicWrite", "Class Name (localized)"="SharedVariableDynamicWrite"}, {"Unique ID string"="16534", "Parent ID string"="16401", "Class Name (unlocalized)"="GenericSubVI", "Class Name (localized)"="GenericSubVI"}, {"Unique ID string"="16535", "Parent ID string"="16429", "Class Name (unlocalized)"="InRangeAndCoerce", "Class Name (localized)"="InRangeAndCoerce"}, {"Unique ID string"="16536", "Parent ID string"="16426", "Class Name (unlocalized)"="RegionTunnel", "Class Name (localized)"="RegionTunnel"}, {"Unique ID string"="16538", "Parent ID string"="16482", "Class Name (unlocalized)"="TypedRefNumConstant", "Class Name (localized)"="TypedRefNumConstant"}, {"Unique ID string"="16539", "Parent ID string"="16538", "Class Name (unlocalized)"="DataValRefNumConstant", "Class Name (localized)"="DataValRefNumConstant"}, {"Unique ID string"="16540", "Parent ID string"="16421", "Class Name (unlocalized)"="TextBaseNode", "Class Name (localized)"="TextBaseNode"}, {"Unique ID string"="16541", "Parent ID string"="16540", "Class Name (unlocalized)"="ExpressionNode", "Class Name (localized)"="ExpressionNode"}, {"Unique ID string"="16542", "Parent ID string"="16410", "Class Name (unlocalized)"="RegisterForEvents", "Class Name (localized)"="RegisterForEvents"}, {"Unique ID string"="16543", "Parent ID string"="16404", "Class Name (unlocalized)"="TargetStructureNode", "Class Name (localized)"="TargetStructureNode"}, {"Unique ID string"="16546", "Parent ID string"="16406", "Class Name (unlocalized)"="RaceStructureNode", "Class Name (localized)"="RaceStructureNode"}, {"Unique ID string"="16545", "Parent ID string"="16404", "Class Name (unlocalized)"="ClosureStructureNode", "Class Name (localized)"="ClosureStructureNode"}, {"Unique ID string"="16544", "Parent ID string"="16517", "Class Name (unlocalized)"="InPlaceVariantAttributeNode", "Class Name (localized)"="InPlaceVariantAttributeNode"}, {"Unique ID string"="16547", "Parent ID string"="16463", "Class Name (unlocalized)"="ExternalEditorWizard", "Class Name (localized)"="ExternalEditorWizard"}, {"Unique ID string"="16548", "Parent ID string"="16517", "Class Name (unlocalized)"="InPlaceMapNode", "Class Name (localized)"="InPlaceMapNode"}, {"Unique ID string"="16549", "Parent ID string"="16410", "Class Name (unlocalized)"="BuildSetNode", "Class Name (localized)"="BuildSetNode"}, {"Unique ID string"="16550", "Parent ID string"="16410", "Class Name (unlocalized)"="BuildMapNode", "Class Name (localized)"="BuildMapNode"}, {"Unique ID string"="16551", "Parent ID string"="16410", "Class Name (unlocalized)"="AssertStructuralTypeMismatchNode", "Class Name (localized)"="AssertStructuralTypeMismatchNode"}, {"Unique ID string"="16552", "Parent ID string"="16386", "Class Name (unlocalized)"="SetConstant", "Class Name (localized)"="SetConstant"}, {"Unique ID string"="16553", "Parent ID string"="16386", "Class Name (unlocalized)"="MapConstant", "Class Name (localized)"="MapConstant"}]
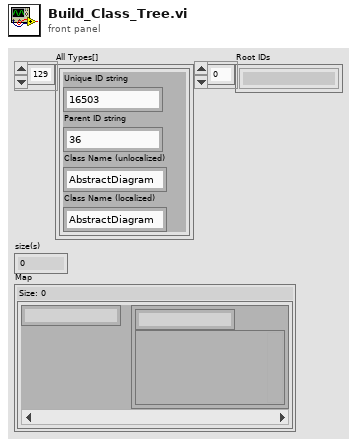
[diagram p1: front panel]
types:
  T1 = typedef "ASC_ArrayOfUniqueIDStringParentIDStringName.ctl" = T2[]
  T2 = typedef "ASC_UniqueIDStringParentIDStringName.ctl" = cluster{"Unique ID string":string, "Parent ID string":string, "Class Name (unlocalized)":string, "Class Name (localized)":string}
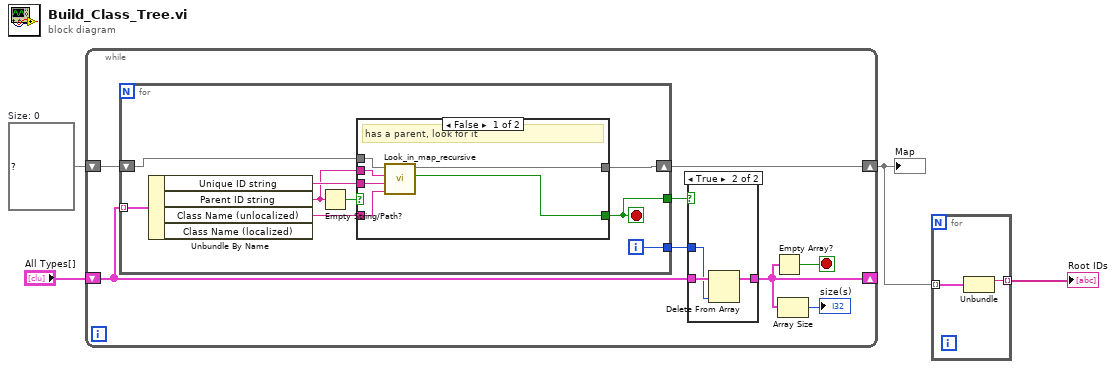
[diagram p0: block diagram]
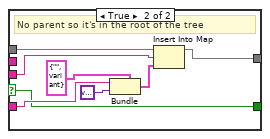
[diagram p3: hidden frame]
diagram:
  w3 = map{string, cluster{string, variant}} {}  # Size: 0
  n1 = while {
    shift-right: [w9] -> _
    shift-left: "All Types[]" -> [w11]
    shift-right: [w7] -> w2
    shift-left: w3 -> [w12]
    stop <- w10 stop-if-true
    n2 = for {
      tunnel: w11 -> [w25] mode=indexing
      shift-right: [w22] -> w7
      shift-left: w12 -> [w23]
      tunnel: [w18] -> w6
      tunnel: [w17] -> w5
      i -> [w17]
      stop <- w18 stop-if-true
      n3 = Unbundle By Name(w25) -> ("Unique ID string"=w21:string, "Parent ID string"=w19:string, "Class Name (unlocalized)"=w20:string)  [unwired: 1 out]
      n4 = Empty String/Path?(string/path=w19) -> (empty?=w24:bool)
      n5 = case shown="False" w24 {
        selector: w24 -> [_ w32]
        tunnel: w23 -> [w31 w39]
        tunnel: [w27 w38] -> w22
        tunnel: w21 -> [w29 w37]
        tunnel: w20 -> [w28 w34]
        tunnel: [w26 w32] -> w18
        tunnel: w19 -> [w30 _]
        frame False {
          # "has a parent, look for it"
          n6 = call "Look_in_map_recursive.vi"("Child Name"=w28, "Child ID"=w29, "Parent ID string"=w30, "Map"=w31) -> ("Parent in Maps"=w26:bool, "Map Out"=w27:map{string, cluster{string, variant}})  [unwired: 6 in]
        }
        frame True {
          # "No parent so it's in the root of the tree"
          n7 = Bundle(cluster=cluster{string, variant} {"", variant} ("value"), w34, variant) -> (w35:cluster{string, variant})
          n8 = Insert Into Map(map in=w39, key=w37, value=w35) -> (map out=w38:map{string, cluster{string, variant}})  [unwired: 2 out]
        }
      }
    }
    n9 = case shown="True" w6 {
      tunnel: w11 -> [w13 w16]
      tunnel: [w13 w15] -> w9
      tunnel: w5 -> [_ w14]
      frame False {
      }
      frame True {
        n10 = Delete From Array(array=w16, index=w14) -> (array with subset deleted=w15:T1)  [unwired: 1 in, 1 out]
      }
    }
    n11 = Empty Array?(array=w9) -> (empty?=w10:bool)
    n12 = Array Size(array=w9) -> (size(s)=→"size(s)":i32)
  }
  "Map" <- w2
  n13 = for {
    tunnel: w2 -> [w41] mode=indexing
    tunnel: [w40] -> w1 mode=indexing
    n14 = Unbundle(w41) -> (w40:string)  [unwired: 1 out]
  }
  "Root IDs" <- w1
